vi "Configuration Error Checker.vi"(8 "error in":errorcluster, 11 "Device DDS Communications in":refnum<class "Device DDS Communications.lvclass">) -> (0 "error out":errorcluster, 3 "Device DDS Communications out":refnum<class "Device DDS Communications.lvclass">)   [LabVIEW 2018, in "Device DDS Communications Framework.lvlib" / "Device DDS Communications.lvclass"]
uses:
  Device DDS Communications.lvclass
  C:/Users/Administrator/Desktop/2018LabVIEW EMS/EMS Generic Actor/EMS Generic/EMS Generic.lvclass
  EMS Generic Actor/EMS Generic/EMS Generic.lvclass
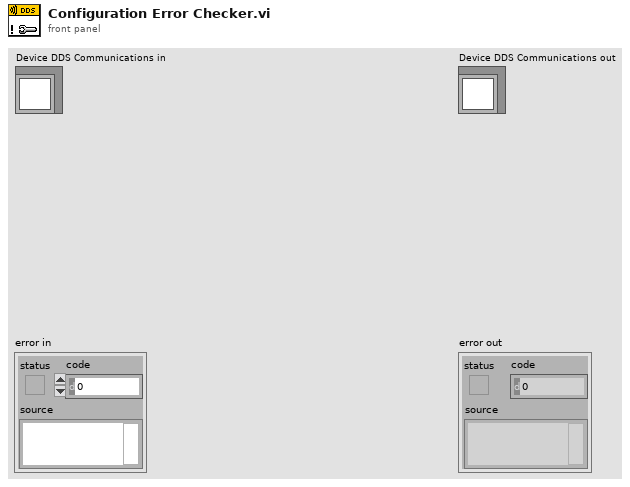
[diagram p1: front panel]
types:
  T1 = typedef "CSEISMIC DDS.lvlib/CSEISMIC DDS.lvclass/DeviceID.ctl" = string
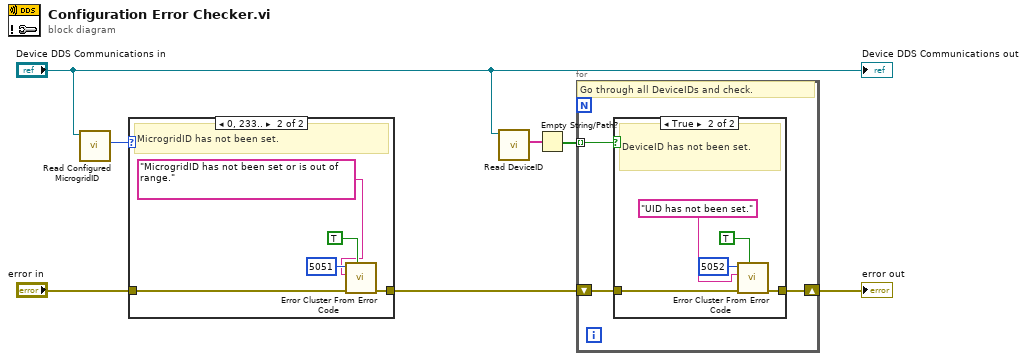
[diagram p0: block diagram]
diagram:
  n1 = call "Read Configured MicrogridID.vi"("EMS Generic in"="Device DDS Communications in") -> ("Microgrid ID"=w2:u8)  [unwired: 8 in, 2 out]
  n2 = case shown="0, 233.." w2 {
    tunnel: "error in" -> [w8 w13]
    tunnel: [w8 w12] -> w5
    frame 1..232 {
      # "MicrogridID has been set."
    }
    frame 0, 233.. {
      # "MicrogridID has not been set."
      n3 = call <vilib>:"Error Cluster From Error Code.vi"("show call chain? (False)"=TRUE, "error in (no error)"=w13, "error message (\"\")"="MicrogridID has not been set or is out of range." ("format string"), "error code (0)"=5051) -> ("error out"=w12:errorcluster)  [unwired: 5 in]
    }
  }
  n4 = call-dynamic "Read DeviceID.vi"("Device DDS Communications in"="Device DDS Communications in") -> ("DeviceID"=w3:T1[])  [unwired: 9 in, 1 out]
  n5 = Empty String/Path?(string/path=w3) -> (empty?=w6:bool[])
  n6 = for {
    tunnel: w6 -> [w16] mode=indexing
    shift-right: [w14] -> w4
    shift-left: w5 -> [w15]
    # "Go through all DeviceIDs and check."
    n7 = case shown="True" w16 {
      tunnel: w15 -> [w17 w22]
      tunnel: [w17 w21] -> w14
      frame False {
        # "DeviceID has been set."
      }
      frame True {
        # "DeviceID has not been set."
        n8 = call <vilib>:"Error Cluster From Error Code.vi"("show call chain? (False)"=TRUE, "error in (no error)"=w22, "error message (\"\")"="UID has not been set." ("format string"), "error code (0)"=5052) -> ("error out"=w21:errorcluster)  [unwired: 5 in]
      }
    }
  }
  "error out" <- w4
  "Device DDS Communications out" <- "Device DDS Communications in"
